vi "Controller Write Outputs.vi"(0 "PS Setpoint Variables":refnum<k21>[](array[refnum]), 1 "PS ON-OFF Variables":refnum<k21>[](array[refnum]), 2 "PS Enable Variables":refnum<k21>[](array[refnum]), 3 "PS Setpoints":dbl[](array[numeric]), 4 "PS ON-OFF (per PS Rack)":u8[](array[numeric]), 5 "error in (no error)":errorcluster) -> (19 "error out":errorcluster)   [LabVIEW 2011, in "Controller VIs.lvlib"]
doc: "Writes all output variables to Actuation chassis."
uses:
  Controller VIs.lvlib
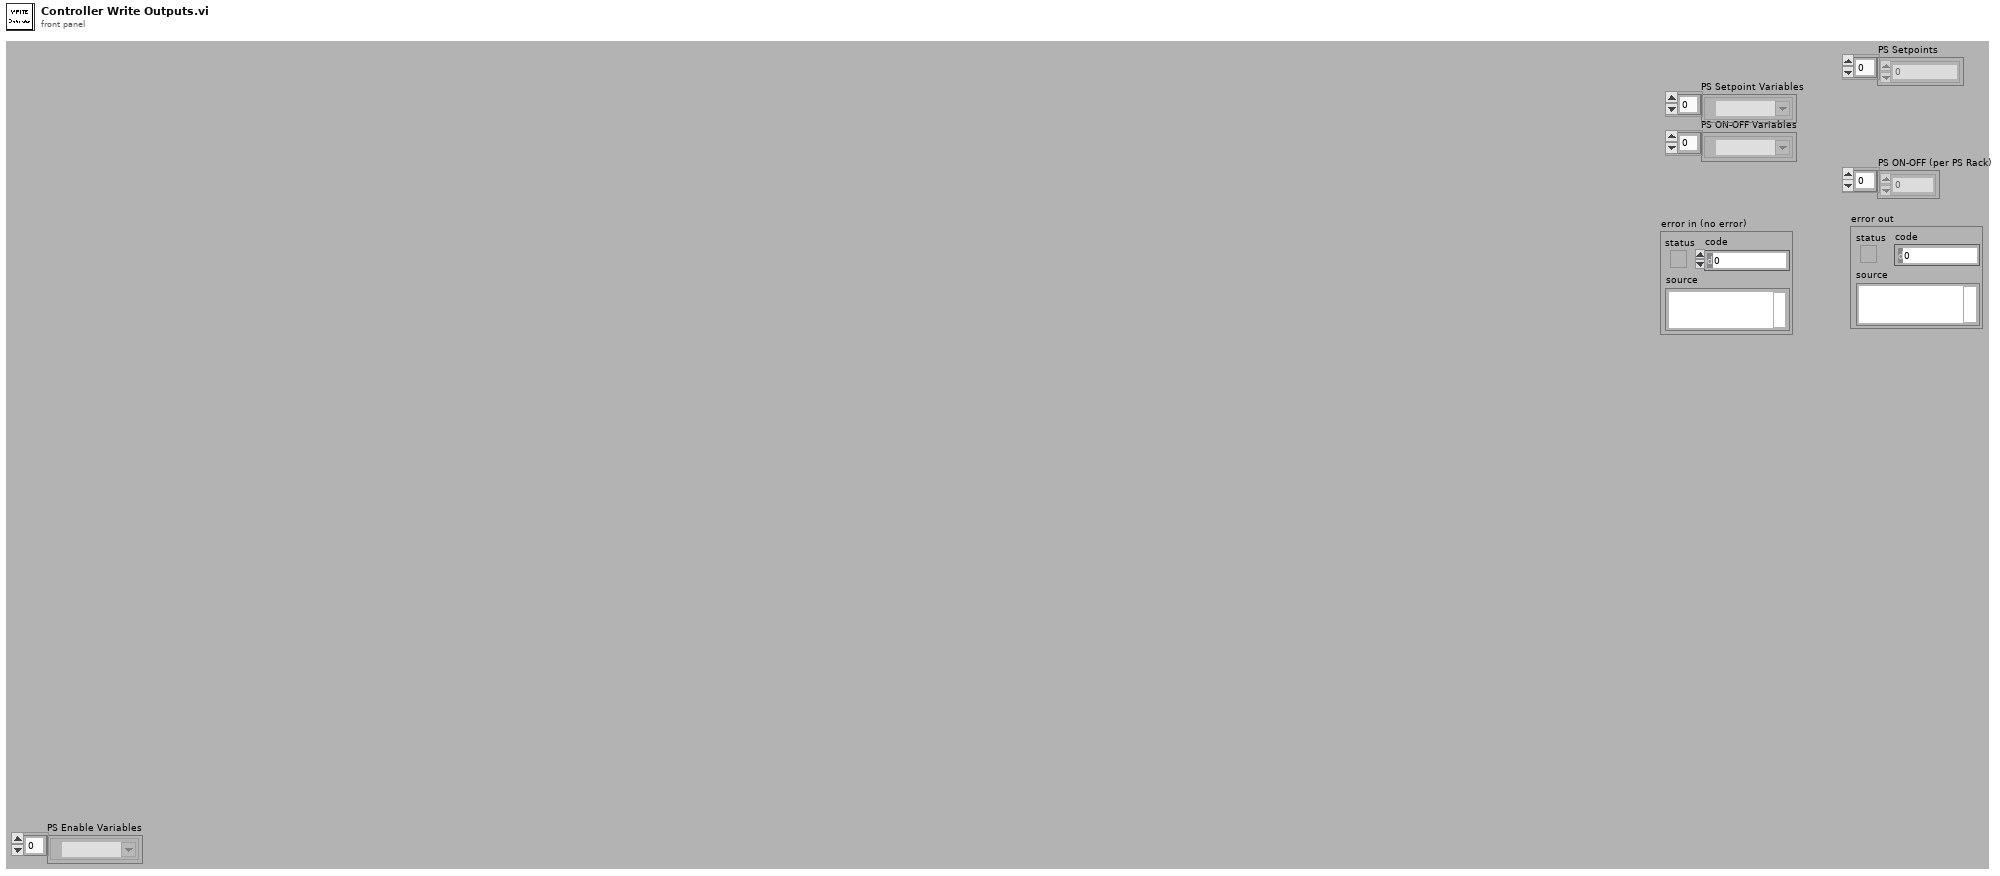
[diagram p1: front panel]
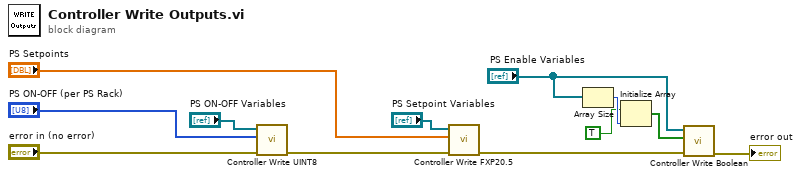
[diagram p0: block diagram]
diagram:
  n1 = call "Controller Write UINT8.vi"("error in (no error)"="error in (no error)", "Values"="PS ON-OFF (per PS Rack)", "Variables"="PS ON-OFF Variables") -> ("error out"=w9:errorcluster)  [unwired: 8 in]
  n2 = call "Controller Write FXP20.5.vi"("Error In"=w9, "Values"="PS Setpoints", "Variables"="PS Setpoint Variables") -> ("Error Out"=w2:errorcluster)  [unwired: 8 in]
  n3 = Array Size(array="PS Enable Variables") -> (size(s)=w6:i32)
  n4 = Initialize Array(TRUE, w6) -> (w5:bool[])
  n5 = call "Controller Write Boolean.vi"("Error In"=w2, "Values"=w5, "Variables"="PS Enable Variables") -> ("Error Out"=→"error out":errorcluster)  [unwired: 8 in]
